vi "DeleteSymbolsInDir.vi"(8 "error in (no error)":errorcluster, 10 "pattern":string="开发环境 *", 11 "dup path":path) -> (0 "error in (no error) (dup)":errorcluster, 3 "dup path (dup)":path)   [LabVIEW 2017, in "application.lvlib" / "application.lvclass"]
uses:
  application.lvclass
panel:
  out "file names":string[](array[string])
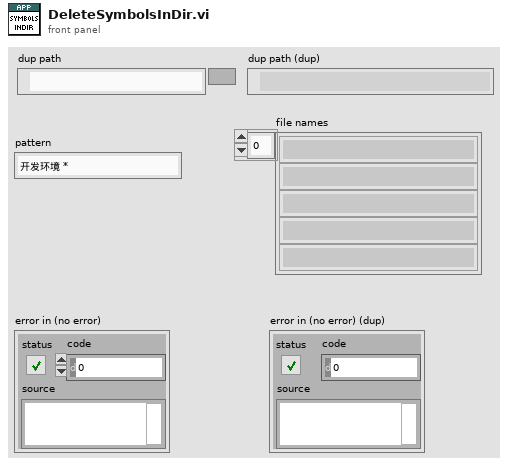
[diagram p1: front panel]
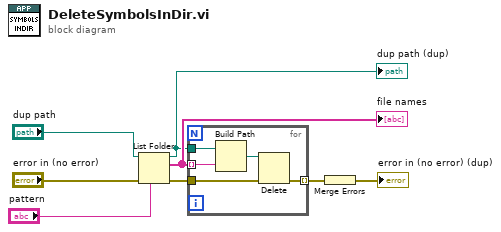
[diagram p0: block diagram]
diagram:
  n1 = List Folder(path="dup path", pattern="pattern", error in="error in (no error)") -> (path out=w3:path, filenames=w4:string[], error out=w5:errorcluster)  [unwired: 1 in, 1 out]
  "dup path (dup)" <- w3
  "file names" <- w4
  n2 = for {
    tunnel: w4 -> [w12] mode=indexing
    tunnel: w5 -> [w13]
    tunnel: w3 -> [w11]
    tunnel: [w9] -> w2 mode=indexing
    n3 = Build Path(base path=w11, name or relative path=w12) -> (appended path=w10:path)
    n4 = Delete(path (use dialog)=w10, error in=w13) -> (error out=w9:errorcluster)  [unwired: 3 in, 2 out]
  }
  n5 = Merge Errors(w2) -> (→"error in (no error) (dup)":errorcluster)
